vi "Script Select UI - DBL Array Example.vi"(7 "Server Alias":string) -> ()   [LabVIEW 2013]
doc: "This VI allows the user to select a script to run on the Python side."
uses:
  LabVIEW Core/TS.lvlib
panel:
  in  "Double Array to pass":dbl[](array[numeric])
  in  "Python Script to Run":path=path "C:/Projects/IN110094 Python LabVIEW Interface/Python Core/Test Scripts"
  in  "Cancel Button":bool
  in  "OK Button":bool
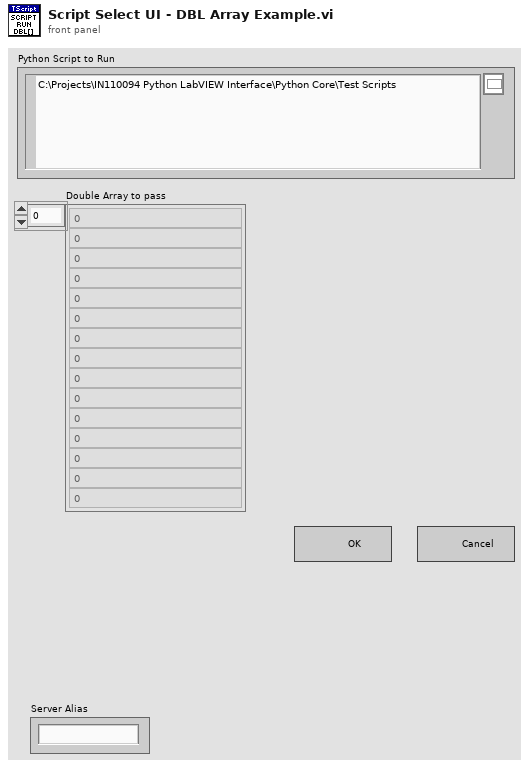
[diagram p1: front panel]
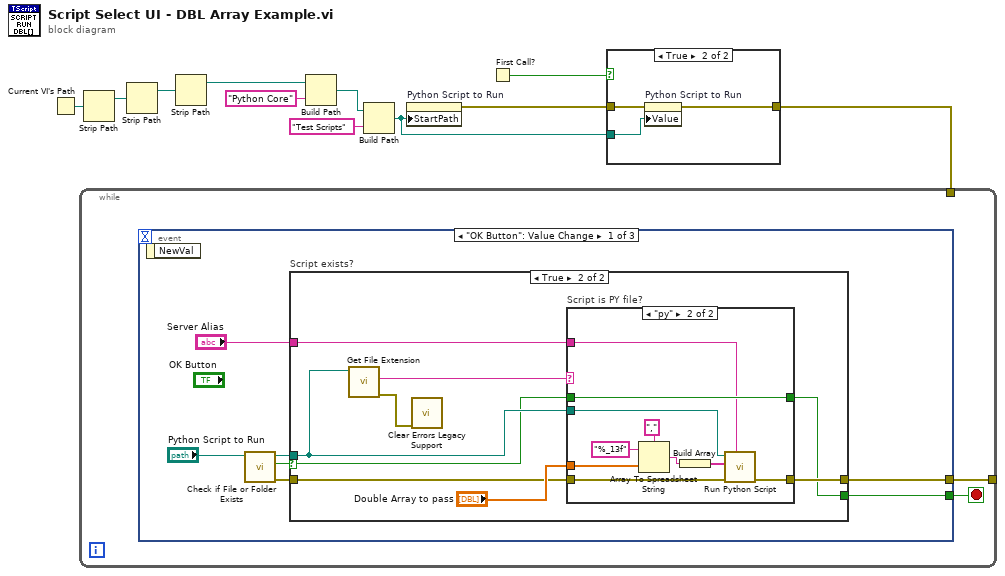
[diagram p0: block diagram]
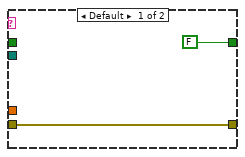
[diagram p4: hidden frame]
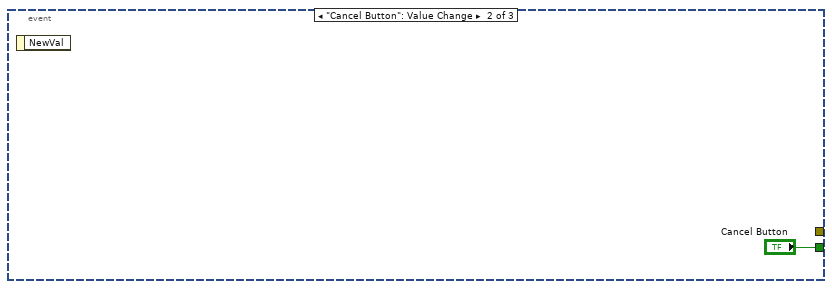
[diagram p5: hidden frame]
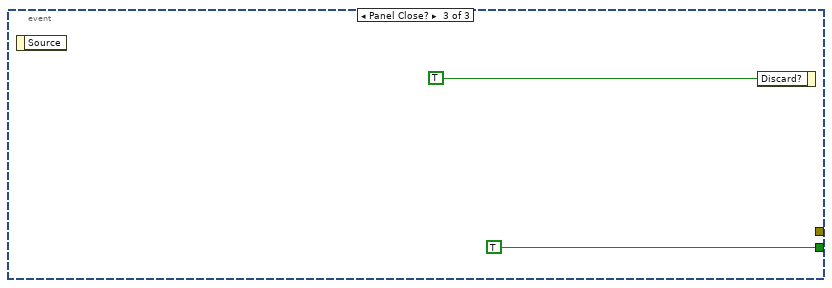
[diagram p6: hidden frame]
diagram:
  n1 = Current VI's Path() -> (path=w8:path)
  n2 = Strip Path(path=w8) -> (stripped path=w10:path)  [unwired: 1 out]
  n3 = Strip Path(path=w10) -> (stripped path=w11:path)  [unwired: 1 out]
  n4 = Strip Path(path=w11) -> (stripped path=w5:path)  [unwired: 1 out]
  n5 = Build Path(base path=w5, name or relative path="Python Core") -> (appended path=w6:path)
  n6 = Build Path(base path=w6, name or relative path="Test Scripts") -> (appended path=w3:path)
  n7 = property on="Python Script to Run" class="Path"("StartPath"=w3) -> (error out=w4:errorcluster)  [unwired: 2 in, 1 out]
  n8 = First Call?() -> (First Call?: T/F=w1:bool)
  n9 = case shown="True" w1 {
    tunnel: w4 -> [w12 w15]
    tunnel: w3 -> [_ w14]
    tunnel: [w12 w13] -> w2
    frame False {
    }
    frame True {
      n10 = property on="Python Script to Run" class="Path"(error in=w15, "Value"=w14) -> (error out=w13:errorcluster)  [unwired: 1 in, 1 out]
    }
  }
  n11 = while {
    tunnel: [w16] -> _
    tunnel: w2 -> [_]
    stop <- w17 stop-if-true
    n12 = event shown="[0] \"OK Button\": Value Change" {
      selector: _ -> [_ _ _]
      dyn-events: _ -> [_ _ _]
      timeout: _ -> [_ _ _]
      tunnel: [w21 "Cancel Button" TRUE ("Cancel Button")] -> w17
      tunnel: [w20 _ _] -> w16
      event "OK Button": Value Change {
        n13 = event-data() -> ()  [unwired: 1 in, 1 out]
        n14 = call <vilib>:"Check if File or Folder Exists.vi"("path"="Python Script to Run") -> ("error out"=w19:errorcluster, "file or folder exists?"=w23:bool, "dup path"=w22:path)  [unwired: 8 in]
        n15 = case "Script exists?" shown="True" w23 {
          selector: w23 -> [w25 w27]
          tunnel: w22 -> [_ w31]
          tunnel: [w25 w28] -> w21
          tunnel: [_ w33] -> w20
          tunnel: w19 -> [_ w32]
          tunnel: "Server Alias" -> [_ w26]
          frame False {
          }
          frame True {
            n16 = call <vilib>:"Get File Extension.vi"("file"=w31) -> ("error out"=w29:errorcluster, "lowercase file extension"=w30:string)  [unwired: 6 in, 3 out]
            n17 = call "Clear Errors Legacy Support.vi"("error in (no error)"=w29) -> ()  [unwired: 5 in, 2 out]
            n18 = case "Script is PY file?" shown="\"py\"" w30 {
              tunnel: "Double Array to pass" -> [_ w43]
              tunnel: [w36 w46] -> w33
              tunnel: w32 -> [w36 w42]
              tunnel: w31 -> [_ w45]
              tunnel: [FALSE w44] -> w28
              tunnel: w27 -> [_ w44]
              tunnel: w26 -> [_ w37]
              frame Default {
              }
              frame "py" {
                n19 = Array To Spreadsheet String(delimiter (Tab)=",", array=w43, 3:"%_13f" ("format string")) -> (spreadsheet string=w39:string)
                n20 = Build Array(w39) -> (w38:string[])
                n21 = call "Run Python Script.vi"("Server Alias"=w37, "error in (no error)"=w42, "Script Arguments (Optional)"=w38, "Absolute Python Script Path"=w45) -> ("error out"=w46:errorcluster)  [unwired: 7 in]
              }
            }
          }
        }
      }
      event "Cancel Button": Value Change {
        n22 = event-data() -> ()  [unwired: 1 in, 1 out]
      }
      event Panel Close? {
        n23 = event-data() -> ()  [unwired: 1 in, 1 out]
        n24 = event-data("Discard?"=TRUE) -> ()  [unwired: 1 in, 1 out]
      }
    }
  }
